vi "Update Enum Value.vi"(9 "Value":string, 10 "Tree Tag":string, 11 "Settings In":T1) -> (3 "Settings Out":T1)   [LabVIEW 2024, in "Sequencer with Output Values.lvlib" / "Sequencer with Output Values.lvclass"]
uses:
  Sequencer with Output Values.lvclass
  Params.ctl
  Step Settings.ctl
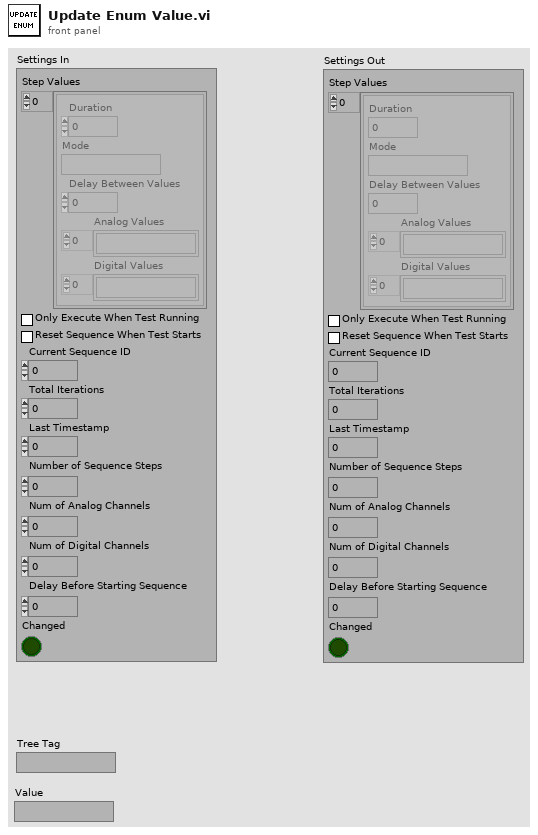
[diagram p1: front panel]
types:
  T1 = typedef "Sequencer with Output Values.lvlib/Sequencer with Output Values.lvclass/Params.ctl" = cluster{"Step Values":T2[], "Only Execute When Test Running":bool, "Reset Sequence When Test Starts":bool, "Current Sequence ID":u32, "Total Iterations":u32, "Last Timestamp":dbl, "Number of Sequence Steps":i32, "Num of Analog Channels":i32, "Num of Digital Channels":i32, "Delay Before Starting Sequence":dbl, "Changed":bool}
  T2 = typedef "Sequencer with Output Values.lvlib/Sequencer with Output Values.lvclass/Step Settings.ctl" = cluster{"Duration":dbl, "Mode":string, "Delay Between Values":dbl, "Analog Values":string[], "Digital Values":string[]}
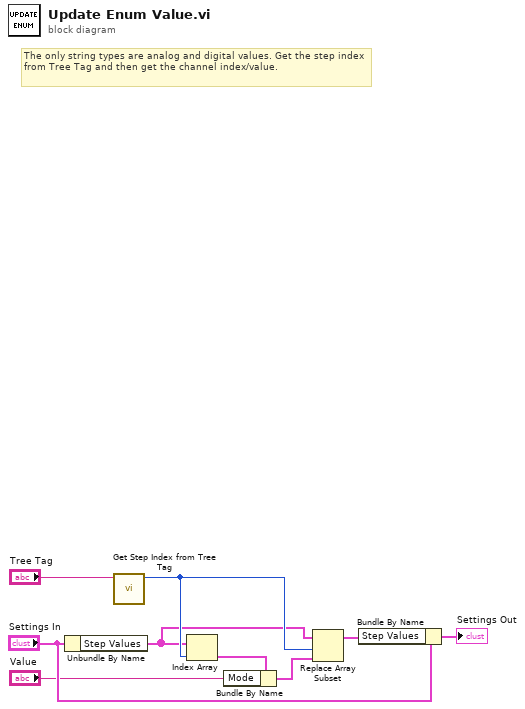
[diagram p0: block diagram]
diagram:
  # "The only string types are analog and digital values. Get the step index from Tree Tag and then get the channel index/value."
  n1 = Unbundle By Name("Settings In") -> ("Step Values"=w7:T2[])
  n2 = call "Get Step Index from Tree Tag.vi"("Tree Tag"="Tree Tag") -> ("Step Index"=w8:i32)  [unwired: 9 in, 1 out]
  n3 = Index Array(array=w7, index=w8) -> (element=w3:T2)
  n4 = Bundle By Name(cluster=w3, "Mode"="Value") -> (w1:T2)
  n5 = Replace Array Subset(array=w7, new element=w1, index=w8) -> (w5:T2[])
  n6 = Bundle By Name(cluster="Settings In", "Step Values"=w5) -> (→"Settings Out":T1)
